vi "zero pos abs.vi"(8 "error in (no error)":errorcluster, 10 "velocity":dbl, 11 "Encoder":T1) -> (0 "error out":errorcluster)   [LabVIEW 2023]
uses:
  <vilib>/Rock Robotics/WPI/ThirdParty/Phoenix-LabVIEW/CANCoder/Controls/CTRE_Phoenix_CANcoder_DeviceRef.ctl
  <vilib>/Rock Robotics/WPI/ThirdParty/Phoenix-LabVIEW/CANCoder/Set/CTRE_Phoenix_CANcoder_SetPositionToAbsolute.vi
panel:
  in  "velocity\ndeadband":dbl=0.01 format="%#_13g"
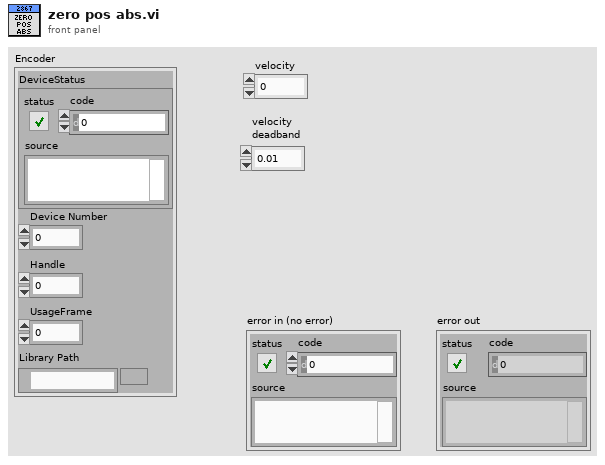
[diagram p1: front panel]
types:
  T1 = typedef "CTRE_Phoenix_CANcoder_DeviceRef.ctl" = cluster{"DeviceStatus":errorcluster, "Device Number":u8, "Handle":u64, "UsageFrame":u32, "Library Path":path}
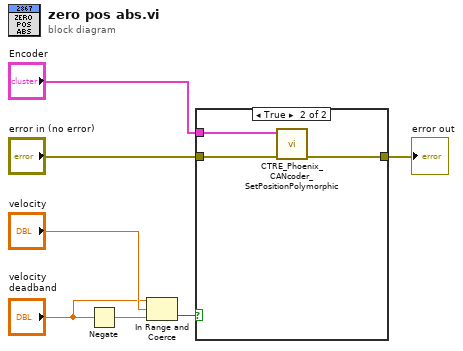
[diagram p0: block diagram]
diagram:
  n1 = Negate(x="velocity\ndeadband") -> (-x=w4:dbl)
  n2 = In Range and Coerce(upper limit="velocity\ndeadband", x="velocity", lower limit=w4) -> (In Range?=w5:bool)  [unwired: 1 out]
  n3 = case shown="True" w5 {
    tunnel: "Encoder" -> [_ w11]
    tunnel: [w8 w10] -> w2
    tunnel: "error in (no error)" -> [w8 w9]
    frame False {
    }
    frame True {
      n4 = call-poly <vilib>:"CTRE_Phoenix_CANcoder_SetPositionPolymorphic.vi"("error in (no error)"=w9, "CTRE_CANcoder_DeviceRef"=w11) -> ("error out"=w10:errorcluster)  [unwired: 8 in, 1 out]
    }
  }
  "error out" <- w2
